vi "ao_dc_voltage.vi"() -> ()   [LabVIEW 2020]
panel:
  in  "Voltage 3":sgl
  in  "Voltage 2":sgl
  in  "Voltage 1":sgl
  out "error out":errorcluster caption="错误输出"
  in  "Voltage 0":sgl
  in  "DevIndex":i32
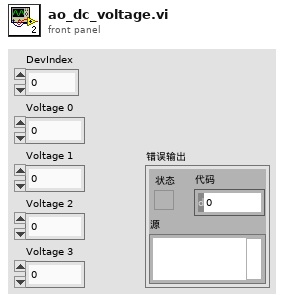
[diagram p1: front panel]
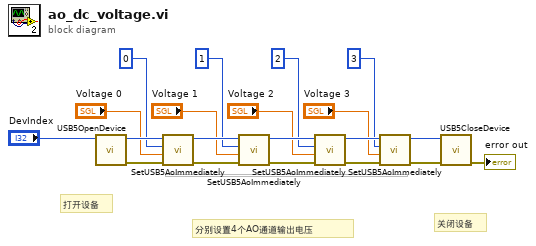
[diagram p0: block diagram]
diagram:
  # "关闭设备"
  # "分别设置4个AO通道输出电压"
  # "打开设备"
  n1 = call "USB5OpenDevice.vi"("DevIndex"="DevIndex") -> ("error out"=w18:errorcluster, "DevIndex Out"=w20:i32)  [unwired: 9 in]
  n2 = call "SetUSB5AoImmediately.vi"("错误输入（无错误）"=w18, "Voltage"="Voltage 0", "Chan"=u8 0, "DevIndex"=w20) -> ("错误输出"=w16:errorcluster, "DevIndex Out"=w15:i32)  [unwired: 6 in]
  n3 = call "SetUSB5AoImmediately.vi"("错误输入（无错误）"=w16, "Voltage"="Voltage 1", "Chan"=u8 1, "DevIndex"=w15) -> ("错误输出"=w11:errorcluster, "DevIndex Out"=w12:i32)  [unwired: 6 in]
  n4 = call "SetUSB5AoImmediately.vi"("错误输入（无错误）"=w11, "Voltage"="Voltage 2", "Chan"=u8 2, "DevIndex"=w12) -> ("错误输出"=w14:errorcluster, "DevIndex Out"=w13:i32)  [unwired: 6 in]
  n5 = call "SetUSB5AoImmediately.vi"("错误输入（无错误）"=w14, "Voltage"="Voltage 3", "Chan"=u8 3, "DevIndex"=w13) -> ("错误输出"=w9:errorcluster, "DevIndex Out"=w10:i32)  [unwired: 6 in]
  n6 = call "USB5CloseDevice.vi"("错误输入（无错误）"=w9, "DevIndex"=w10) -> ("error out"=→"error out":errorcluster)  [unwired: 8 in, 1 out]
